vi "editscenario format Condition.vi"(8 "Index (0)":i32, 11 "POST (empty)":T1) -> (0 "Valid Condition?":bool, 2 "Condition":T2, 3 "POST out":T1)   [LabVIEW 2011]
uses:
  server/database/Scenarios/Conditions/Condition Record.ctl
  server/database/Scenarios/Conditions/Condition Operators.ctl
  ITK EXT/utils/keyedarr.llb/Keyed Array.ctl
  ITK EXT/utils/strutil.llb/Case Matching.ctl
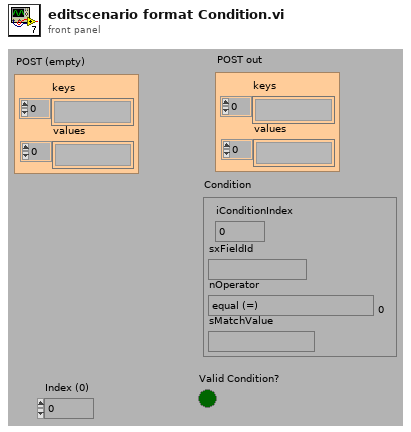
[diagram p1: front panel]
types:
  T1 = typedef "Keyed Array.ctl" = cluster{"keys":string[], "values":string[]}
  T2 = typedef "Condition Record.ctl" = cluster{"iConditionIndex":i32, "sxFieldId":string, "nOperator":T3, "sMatchValue":string}
  T3 = typedef "Condition Operators.ctl" = enum16{"equal (=)", "not equal (\\u2260)", "less than (<)", "less than or equal (\\u2264)", "greater than (>)", "greater than or equal (\\u2265)", "contains", "does not contain"}
  T4 = typedef "Case Matching.ctl" = enum16{"a != A", "a == A", "system"}
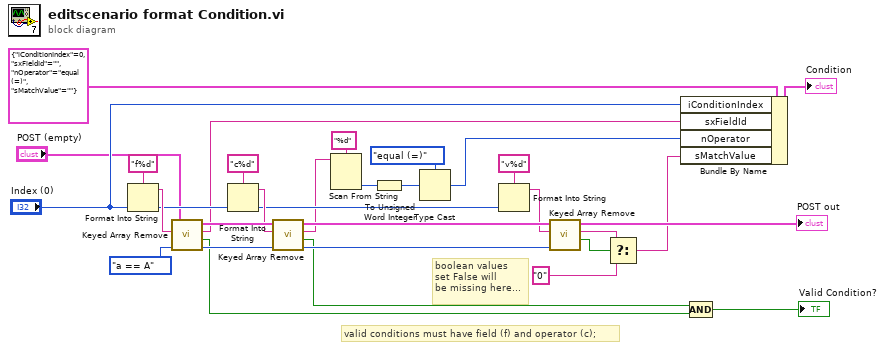
[diagram p0: block diagram]
diagram:
  w26 = Case_Matching."a == A" ("case matching (sensitive)")
  # "valid conditions must have field (f) and operator (c);"
  # "boolean values\nset False will\nbe missing here..."
  n1 = Format Into String(format string="f%d", "Index (0)") -> (resulting string=w22:string)  [unwired: 2 in, 1 out]
  n2 = call "Keyed Array Remove.vi"("case matching (sensitive)"=w26, "key"=w22, "array in"="POST (empty)") -> ("valid key"=w18:bool, "value"=w14:string, "array out"=w28:T1)  [unwired: 2 out]
  n3 = Format Into String(format string="c%d", "Index (0)") -> (resulting string=w21:string)  [unwired: 2 in, 1 out]
  n4 = call "Keyed Array Remove.vi"("case matching (sensitive)"=w26, "key"=w21, "array in"=w28) -> ("valid key"=w19:bool, "value"=w12:string, "array out"=w27:T1)  [unwired: 2 out]
  n5 = Scan From String(format string="%d", input string=w12) -> (output 1=w11:i32)  [unwired: 2 in, 4 out]
  n6 = To Unsigned Word Integer(number=w11) -> (unsigned 16bit integer=w9:u16)
  n7 = Type Cast(type=Condition_Operators."equal (=)" ("nOperator"), x=w9) -> (*(type *) &x=w8:T3)
  n8 = Format Into String(format string="v%d", "Index (0)") -> (resulting string=w20:string)  [unwired: 2 in, 1 out]
  n9 = call "Keyed Array Remove.vi"("case matching (sensitive)"=w26, "key"=w20, "array in"=w27) -> ("valid key"=w4:bool, "value"=w3:string, "array out"=→"POST out":T1)  [unwired: 2 out]
  n10 = Select(t=w3, s=w4, f="0") -> (s? t:f=w2:string)
  n11 = Bundle By Name(cluster=T2 {"iConditionIndex"=0, "sxFieldId"="", "nOperator"=enum."equal (=)", "sMatchValue"=""} ("Condition"), "iConditionIndex"="Index (0)", "sxFieldId"=w14, "nOperator"=w8, "sMatchValue"=w2) -> (→"Condition":T2)
  n12 = Compound Arithmetic op=AND(w19, w18) -> (→"Valid Condition?":bool)
